vi "Get requst ID or error.vi"(8 "error in (no error)":errorcluster, 11 "IHandleUnsubscribed JSON in":refnum<class "IHandleUnsubscribed JSON.lvclass">) -> (0 "error out":errorcluster, 1 "ErrorOrSuccess":refnum<class "ErrorOrSuccess.lvclass">, 2 "Unsubscription Request ID":u64, 3 "IHandleUnsubscribed JSON out":refnum<class "IHandleUnsubscribed JSON.lvclass">)   [LabVIEW 2020, in "wamplv.lvlib" / "IHandleUnsubscribed JSON.lvclass"]
uses:
  IHandleUnsubscribed JSON.lvclass
  IHandleUnsubscribed JSON.lvclass/IHandleUnsubscribed JSON.ctl
  SerialisedMessages/JSONMessage/WampMessage JSON.lvclass
  Error/ErrorHandler JSON/ErrorHandler JSON.lvclass
  Message loop classes/ErrorOrSuccess JSON/ErrorOrSuccess JSON.lvclass
  <vilib>/Utility/error.llb/Error Cluster From Error Code.vi
  <vilib>/ErrorRing/Error Ring.xnode
  C:/local/wamplv/Private/Message loop classes/ErrorOrSuccess/ErrorOrSuccess.lvclass
  C:/local/wamplv/Private/Message loop classes/ErrorOrSuccess JSON/ErrorOrSuccess JSON.lvclass
  Message loop classes/ErrorOrSuccess/ErrorOrSuccess.lvclass
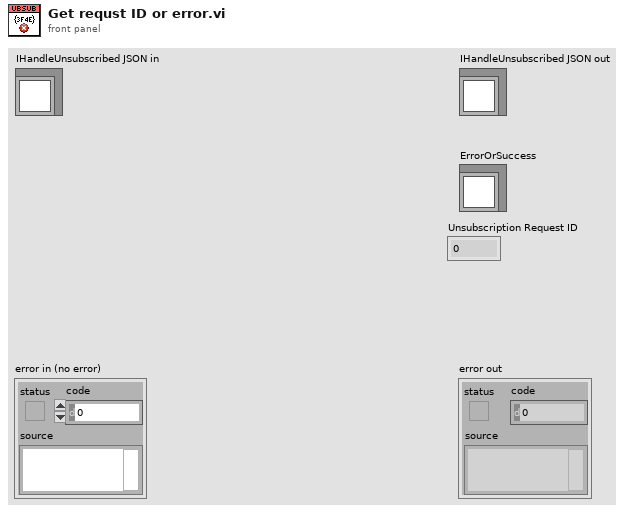
[diagram p1: front panel]
types:
  T1 = typedef "wamplv.lvlib/WAMP Message Codes.ctl" = enum8{"HELLO", "WELCOME", "CHALLENGE", "AUTHENTICATE", "ABORT", "GOODBYE", "ERROR", "PUBLISH", "PUBLISHED", "SUBSCRIBE", "SUBSCRIBED", "UNSUBSCRIBE", "UNSUBSCRIBED", "EVENT", "CALL", "RESULT", "REGISTER", "REGISTERED", "UNREGISTER", "UNREGISTERED", "INVOCATION", "YIELD"}
  T2 = typedef "wamplv.lvlib/Error (JSON).ctl" = cluster{"Request ID":u64, "Message type that caused error":T1, "Error/Abort details (JSON)":T3}
  T3 = typedef "wamplv.lvlib/Error or abort detail (JSON).ctl" = cluster{"Error URI":string, "Error Arguments":string, "Error ArgumentKw":string, "Error Details":string, "Associated LabVIEW Error":errorcluster}
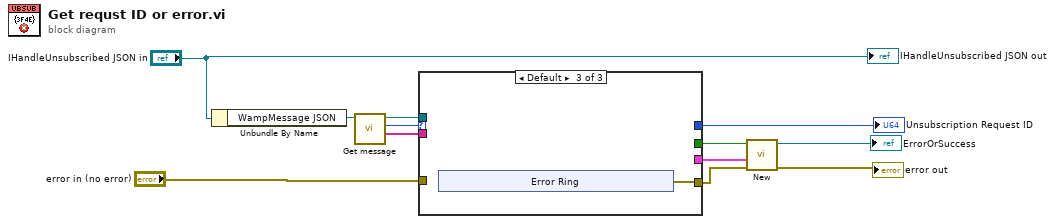
[diagram p0: block diagram]
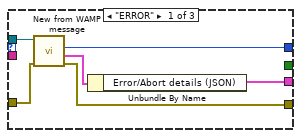
[diagram p2: hidden frame]
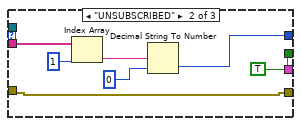
[diagram p3: hidden frame]
diagram:
  n1 = Unbundle By Name("IHandleUnsubscribed JSON in") -> ("WampMessage JSON"=w12:refnum<class "WampMessage JSON.lvclass">)
  n2 = call "Get message.vi"("JSONMessage in"=w12) -> ("<JSON>Elements"=w8:string[], "Message Type"=w10:T1, "JSONMessage out"=w9:refnum<class "WampMessage JSON.lvclass">)  [unwired: 8 in]
  n3 = case shown="Default" w10 {
    tunnel: w9 -> [w18 _ _]
    tunnel: w8 -> [_ w22 _]
    tunnel: [w17 w21 _] -> w7
    tunnel: [w15 _ _] -> w5
    tunnel: [_ TRUE _] -> w4
    tunnel: "error in (no error)" -> [w14 w19 _]
    tunnel: [w13 w19 w26] -> w2
    frame "ERROR" {
      n4 = call "New from WAMP message.vi"("error in (no error)"=w14, "wamplv.lvlib:JSONMessage.lvclass"=w18) -> ("error out"=w13:errorcluster, "Error data (JSON)"=w16:T2, "Request ID"=w17:u64)  [unwired: 6 in, 1 out]
      n5 = Unbundle By Name(w16) -> ("Error/Abort details (JSON)"=w15:T3)
    }
    frame "UNSUBSCRIBED" {
      n6 = Index Array(array=w22, index=1) -> (element=w24:string)
      n7 = Decimal String To Number(string=w24, default (0L)=u64 0) -> (number=w21:u64)  [unwired: 1 in, 1 out]
    }
    frame Default {
      n8 = xnode "Error Ring"() -> ("error out"=w26:errorcluster)
    }
  }
  "Unsubscription Request ID" <- w7
  n9 = call "New.vi"("error in (no error)"=w2, "Error/Abort details (JSON)"=w5, "Success?"=w4) -> ("error out"=→"error out":errorcluster, "ErrorOrSuccess JSON out"=→"ErrorOrSuccess":refnum<class "ErrorOrSuccess JSON.lvclass">)  [unwired: 7 in]
  "IHandleUnsubscribed JSON out" <- "IHandleUnsubscribed JSON in"
